vi "xeva-cooling.vi"(3 "error in (no error)":errorcluster, 4 "xeva-cool-on":bool=TRUE, 5 "xeva-camref":T1) -> (0 "error out":errorcluster, 1 "xeva-cooling":bool)   [LabVIEW 2015]
uses:
  <vilib>/Xenics Infrared Solutions/Xeneth LabVIEW API/VIs/Controls/Camara.ctl
  <vilib>/Xenics Infrared Solutions/Xeneth LabVIEW API/VIs/Property/XC Set Property Value L.vi
  <vilib>/Xenics Infrared Solutions/Xeneth LabVIEW API/Xeneth.lvlib
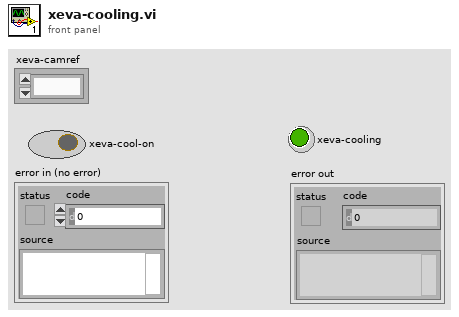
[diagram p1: front panel]
types:
  T1 = typedef "Xeneth.lvlib/Camara.ctl" = refnum<k1>
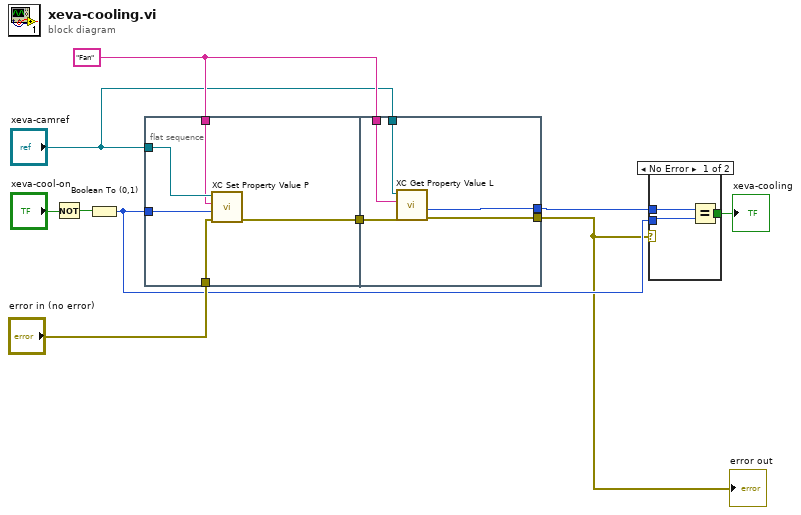
[diagram p0: block diagram]
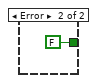
[diagram p2: hidden frame]
diagram:
  w5 = "Fan" ("pPrp")
  n1 = Not(x="xeva-cool-on") -> (.not. x?=w2:bool)
  n2 = Boolean To (0,1)(Boolean=w2) -> (0, 1=w8:i16)
  n3 = flat-sequence {
    tunnel: "xeva-camref" -> [w15]
    tunnel: "error in (no error)" -> [w14]
    tunnel: w5 -> [w12]
    tunnel: w8 -> [w11]
    tunnel: [w13] -> w7
    tunnel: w7 -> [w18]
    tunnel: [w20] -> w3
    tunnel: [w19] -> w6
    tunnel: w5 -> [w17]
    tunnel: "xeva-camref" -> [w16]
    frame #0 {
      n4 = call-poly <vilib>:"XC Set Property Value P.vi"("error in (no error)"=w14, "lValue"=w11, "pPrp"=w12, "Cam Ref"=w15) -> ("error out"=w13:errorcluster)  [unwired: 6 in, 1 out]
    }
    frame #1 {
      n5 = call <vilib>:"XC Get Property Value L.vi"("error in (no error)"=w18, "pPrp"=w17, "Cam Ref"=w16) -> ("error out"=w20:errorcluster, "pValue out"=w19:i32)  [unwired: 6 in, 1 out]
    }
  }
  n6 = case shown="No Error" w3 {
    tunnel: [w23 FALSE] -> w9
    tunnel: w8 -> [w22 _]
    tunnel: w6 -> [w21 _]
    frame No Error {
      n7 = Equal?(x=w21, y=w22) -> (x = y?=w23:bool)
    }
    frame Error {
    }
  }
  "xeva-cooling" <- w9
  "error out" <- w3
